vi "CryoAVC Config Alarms GUI.vi"(11 "Cryo Alarms":T1) -> (3 "Cryo Alarms out":T1)   [LabVIEW 2022 SP3, in "CryoCoolerAVC.lvclass"]
uses:
  CryoCoolerAVC.lvclass
  CryoCoolerAVC.lvclass/CryoCoolerAVC.ctl
  CryoCooler cluster Alarm Settings.ctl
panel:
  in  "Cancel Button":bool
  in  "OK Button":bool
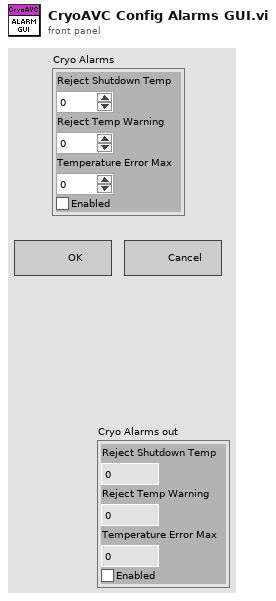
[diagram p1: front panel]
types:
  T1 = typedef "CryoCooler cluster Alarm Settings.ctl" = cluster{"Reject Shutdown Temp":dbl, "Reject Temp Warning":dbl, "Temperature Error Max":dbl, "Enabled":bool}
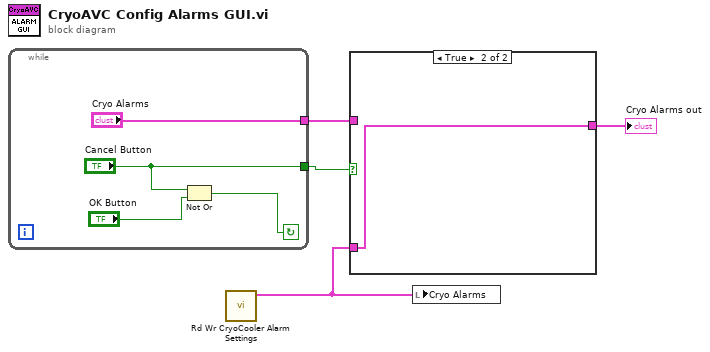
[diagram p0: block diagram]
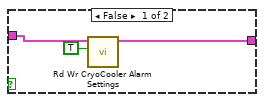
[diagram p2: hidden frame]
diagram:
  n1 = while {
    tunnel: ["Cryo Alarms"] -> w3
    tunnel: ["Cancel Button"] -> w4
    stop <- w7 continue-if-true
    n2 = Not Or(1:"OK Button", 2:"Cancel Button") -> (0:w7:bool)
  }
  n3 = call "Rd Wr CryoCooler Alarm Settings.vi"() -> ("Cryo Alarms out"=w1:T1)  [unwired: 10 in, 1 out]
  n4 = case shown="True" w4 {
    tunnel: w3 -> [w11 _]
    tunnel: [w9 w12] -> w2
    tunnel: w1 -> [_ w12]
    frame False {
      n5 = call "Rd Wr CryoCooler Alarm Settings.vi"("Write? (F:Read)"=TRUE, "Cryo Alarms"=w11) -> ("Cryo Alarms out"=w9:T1)  [unwired: 8 in, 1 out]
    }
    frame True {
    }
  }
  "Cryo Alarms out" <- w2
  n6 = local write "Cryo Alarms"(w1) -> ()
